vi "Configure TS Results.vi"(8 "error in":errorcluster, 11 "DeepU Test Stand in":refnum<class "DeepU Test Stand.lvclass">) -> (0 "error out":errorcluster, 3 "DeepU Test Stand out":refnum<class "DeepU Test Stand.lvclass">)   [LabVIEW 2019, in "Test Stands.lvlib" / "DeepU Test Stand.lvclass"]
uses:
  DeepU Test Stand.lvclass
  Generic Test Stand/Generic Test Stand.lvclass
  Results/Results Method.ctl
  Results/Results.lvlib
  C:/Users/wg/Documents/LV_Projects/test-stand/App/Generic Test Stand/Generic Test Stand.lvclass
  Results/DeepU Results/DeepU Results.lvclass
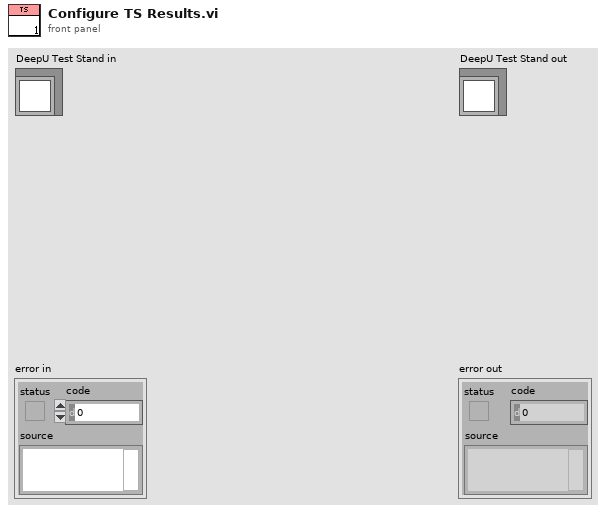
[diagram p1: front panel]
types:
  T1 = typedef "Results.lvlib/Results Method.ctl" = enum16{"Get", "Set"}
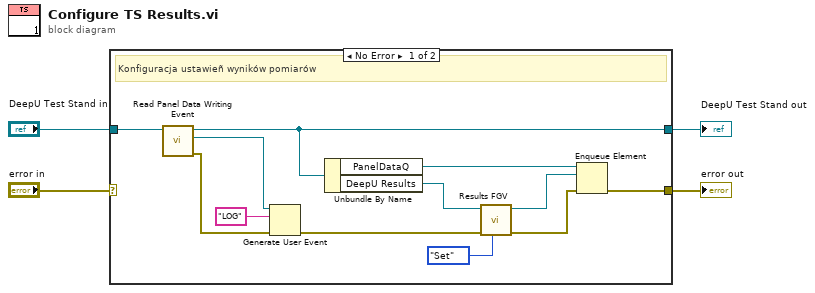
[diagram p0: block diagram]
diagram:
  n1 = case shown="No Error" "error in" {
    selector: "error in" -> [_ w18]
    tunnel: "DeepU Test Stand in" -> [w16 w17]
    tunnel: [w15 w17] -> w3
    tunnel: [w5 w18] -> w4
    frame No Error {
      # "Konfiguracja ustawieñ wyników pomiarów"
      n2 = call "Read Panel Data Writing Event.vi"("Generic Test Stand in"=w16) -> ("error out"=w12:errorcluster, "Panel Data Writing Event"=w14:refnum<user-event>, "Generic Test Stand out"=w15:refnum<class "DeepU Test Stand.lvclass">)  [unwired: 8 in]
      n3 = Generate User Event(user event=w14, event data cluster="LOG" ("event data"), error in=w12) -> (error out=w7:errorcluster)  [unwired: 1 in, 1 out]
      n4 = Unbundle By Name(w15) -> ("PanelDataQ"=w11:refnum<queue>, "DeepU Results"=w9:refnum<class "DeepU Results.lvclass">)
      n5 = call-dynamic "Results FGV.vi"("Method"=Results_Method."Set", "error in"=w7, "LNG Boiling Results in"=w9) -> ("error out"=w8:errorcluster, "LNG Boiling Results out"=w10:refnum<class "DeepU Results.lvclass">)  [unwired: 7 in]
      n6 = Enqueue Element(queue=w11, element=w10, error in (no error)=w8) -> (error out=w5:errorcluster)  [unwired: 1 in, 2 out]
    }
    frame Error {
    }
  }
  "error out" <- w4
  "DeepU Test Stand out" <- w3
